vi "ClosePort.vi"(8 "error in (no error)":errorcluster caption="Fehler (Eingang, kein Fehler)", 11 "MoveoSerial Eingang":refnum<class "MoveoSerial.lvclass">) -> (0 "error out":errorcluster caption="Fehler (Ausgang)", 3 "MoveoSerial Ausgang":refnum<class "MoveoSerial.lvclass">)   [LabVIEW 2019, in "MoveoSerial.lvclass"]
uses:
  MoveoSerial.lvclass
  MoveoSerial.lvclass/MoveoSerial.ctl
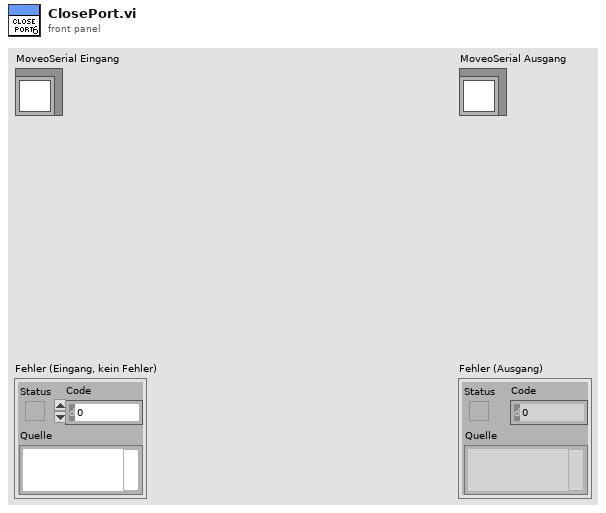
[diagram p1: front panel]
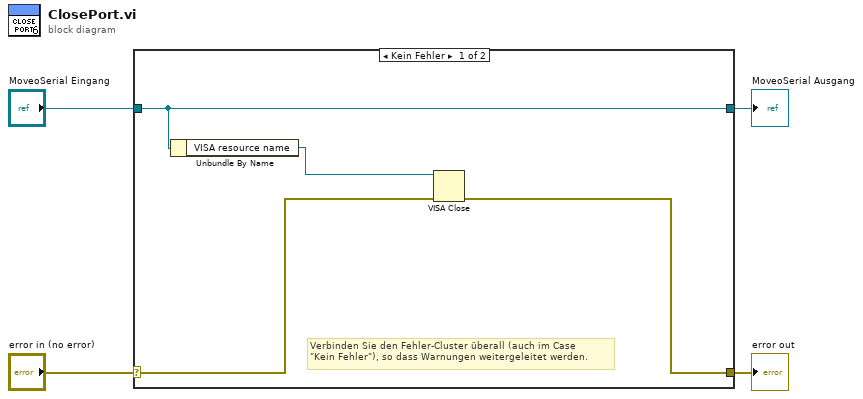
[diagram p0: block diagram]
diagram:
  n1 = case shown="Kein Fehler" "error in (no error)" {
    selector: "error in (no error)" -> [w6 w10]
    tunnel: [w5 w10] -> w3
    tunnel: [w8 w9] -> w1
    tunnel: "MoveoSerial Eingang" -> [w8 w9]
    frame No Error {
      # "Verbinden Sie den Fehler-Cluster überall (auch im Case\n\"Kein Fehler\"), so dass Warnungen weitergeleitet werden."
      n2 = Unbundle By Name(w8) -> ("VISA resource name"=w7:refnum<visa-resource-name>)
      n3 = VISA Close(VISA resource name=w7, error in (no error)=w6) -> (error out=w5:errorcluster)
    }
    frame Error {
    }
  }
  "error out" <- w3
  "MoveoSerial Ausgang" <- w1
